vi "labview.vi"() -> ()   [LabVIEW 2025]
uses:
  <vilib>/sklein/WebView2/Webview2 Lib/WebView2 Control.ctl
  <vilib>/sklein/WebView2/Webview2 Lib/WebView2 Control Object/WebView2 Control.lvclass
  <vilib>/sklein/WebView2/Webview2 Lib/WebView2.lvlib
  <vilib>/sklein/WebView2/Libs/Microsoft.Web.WebView2.WinForms.dll
panel:
  in  "WebView2":T1
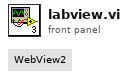
[diagram p1: front panel]
types:
  T1 = typedef "WebView2.lvlib/WebView2 Control.ctl" = refnum<k24>
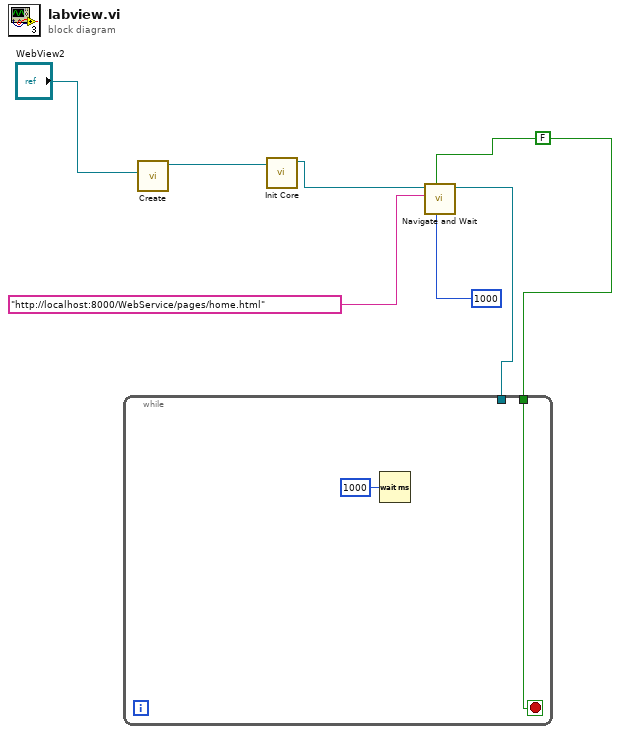
[diagram p0: block diagram]
diagram:
  w1 = FALSE ("html Source (URL)")
  n1 = call <vilib>:"Create.vi"("WebView2 Control"="WebView2") -> ("WebView2 Control out"=w5:refnum<class "WebView2 Control.lvclass">)  [unwired: 9 in, 1 out]
  n2 = call <vilib>:"Init Core.vi"("WebView2 Control in"=w5) -> ("WebView2 Control out"=w2:refnum<class "WebView2 Control.lvclass">)  [unwired: 9 in, 1 out]
  n3 = call <vilib>:"Navigate and Wait.vi"("Timeout (Inf)"=1000, "html Source (URL)"=w1, "Source"="http://localhost:8000/WebService/pages/home.html", "WebView2 Control in"=w2) -> ("WebView2 Control out"=w3:refnum<class "WebView2 Control.lvclass">)  [unwired: 5 in, 2 out]
  n4 = while {
    tunnel: w3 -> [_]
    tunnel: w1 -> [w8]
    stop <- w8 stop-if-true
    n5 = Wait (ms)(milliseconds to wait=u32 1000) -> ()  [unwired: 1 out]
  }
